vi "Raman_Data_Process_subVI.vi"(11 "Spectra Array":cluster{i32[], i32[]}[](array[cluster])) -> (1 "Product Peak Area Trace":i32(graph), 2 "Product Peak Area":i32, 3 "Product Spectrum":cluster{i32[], i32[]}(graph), 4 "Spectrum Length":i32, 5 "Product Peak Height":i32)   [LabVIEW 2015]
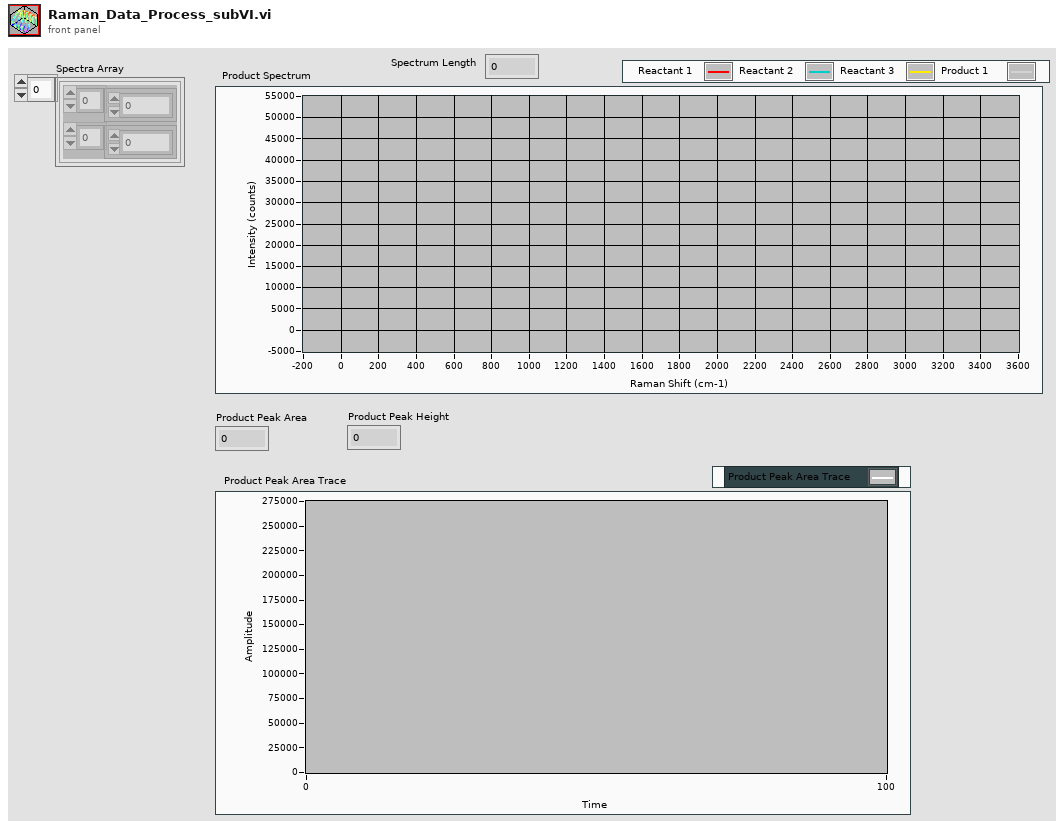
[diagram p1: front panel]
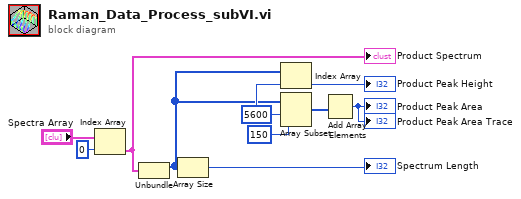
[diagram p0: block diagram]
diagram:
  w3 = 5600 ("index")
  n1 = Index Array(array="Spectra Array", index=0) -> (element=w6:cluster{i32[], i32[]})
  "Product Spectrum" <- w6
  n2 = Unbundle(w6) -> (w2:i32[])  [unwired: 1 out]
  n3 = Array Size(array=w2) -> (size(s)=→"Spectrum Length":i32)
  n4 = Index Array(array=w2, index=w3) -> (element=→"Product Peak Height":i32)
  n5 = Array Subset(array=w2, index=w3, length=150) -> (w9:i32[])
  n6 = Add Array Elements(numeric array=w9) -> (sum=→"Product Peak Area" →"Product Peak Area Trace":i32)
